vi "GET Mouse State.vi"(8 "Error In":errorcluster) -> (0 "Error Out":errorcluster, 3 "Mouse State Out":T1)   [LabVIEW 2014]
uses:
  Controls/GMap Mouse States.ctl
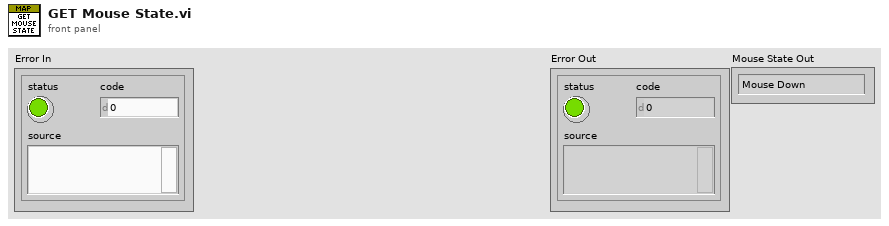
[diagram p1: front panel]
types:
  T1 = typedef "GMap Mouse States.ctl" = enum16{"Mouse Down", "Mouse Up"}
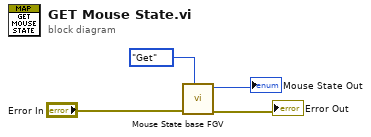
[diagram p0: block diagram]
diagram:
  n1 = call "Mouse State base FGV .vi"("Method"=enum16{"Get", "Set"}."Get", "Error In"="Error In") -> ("Error Out"=→"Error Out":errorcluster, "Mouse State Out"=→"Mouse State Out":T1)  [unwired: 8 in]
